vi "Main.vi"() -> ()   [LabVIEW 2013]
doc: "Use this template to build a simple state machine design pattern. Each state executes code and determines which state to transition to."
uses:
  controls/MainState.ctl
  controls/MainData.ctl
  <vilib>/Utility/file.llb/Read From Spreadsheet File (DBL).vi
panel:
  out "File Path":path
  in  "Binner":bool
  in  "Iteration Start":bool
  in  "Iteration Pause":bool
  in  "Program Stop":bool
  in  "Settings":bool
  in  "Open":bool
  out "Error Chart":dbl(graph)
  out "Spectral Signal":cluster{"X":dbl, "Y":dbl}[](graph)
  out "Temporal Signal":cluster{"X":dbl, "Y":dbl}[](graph)
  out "Retrieved Trace":dbl[][](graph)
  out "Original Trace":dbl[][](graph)
  # "These controls have associated \"Value Changed\" events configured in the Event Structure on the diagram.\n\nReplace them (and reconfigure the Event Structure) with the controls you need for your application."
  # "This template is for the Simple State Machine design pattern.\n\nSee the block diagram for more information on how to use this template."
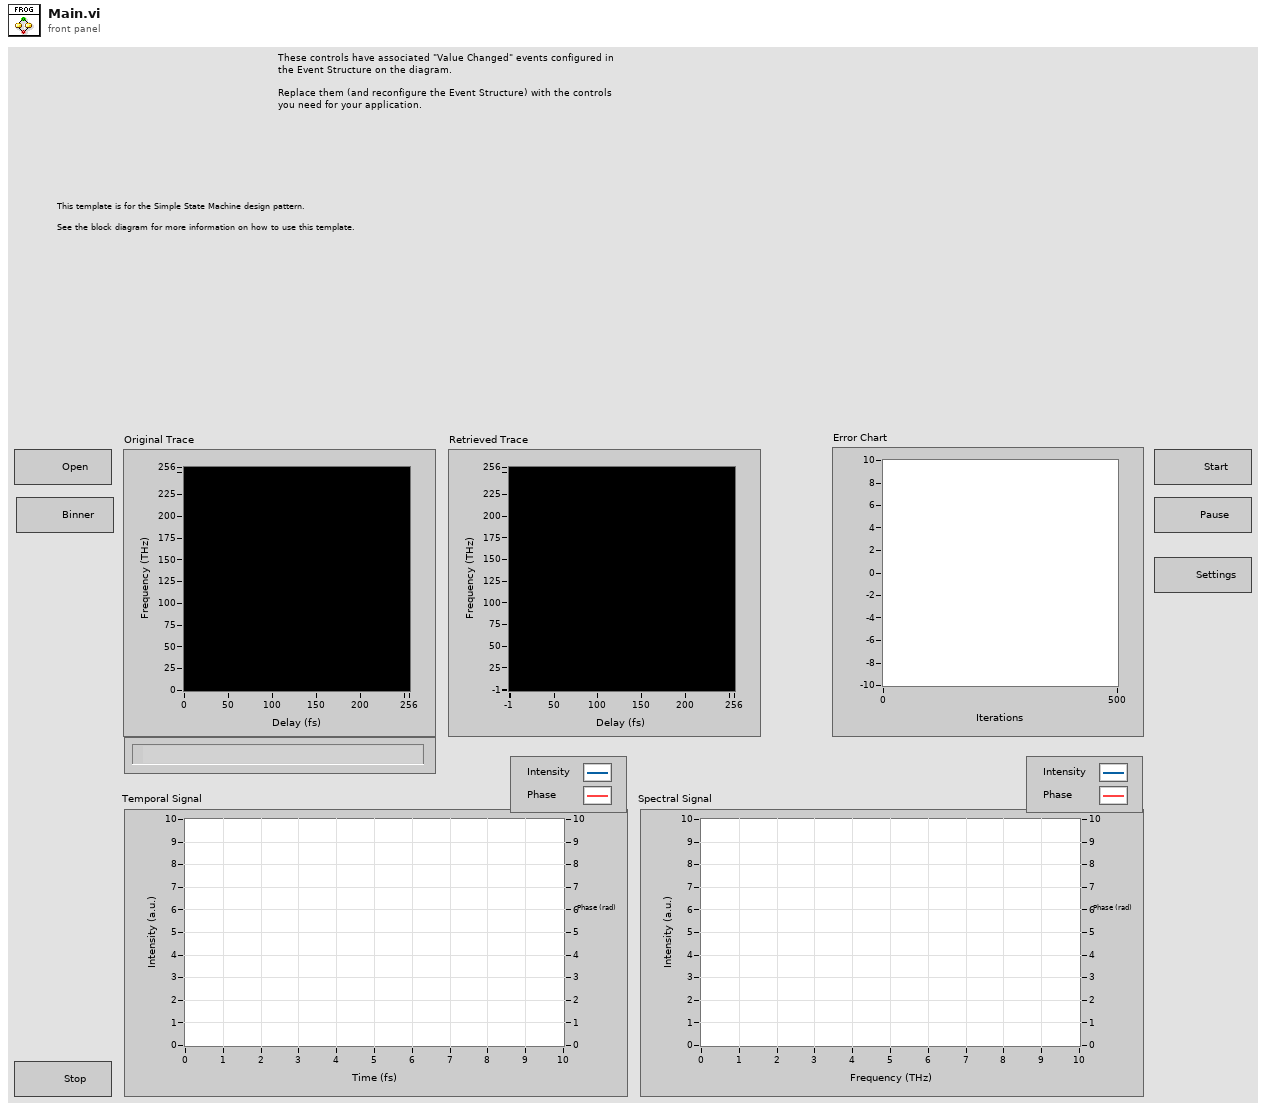
[diagram p1: front panel]
types:
  T1 = typedef "MainData.ctl" = cluster{"Template Trace":dbl[][], "Retrieved Trace":cdb[][], "Spectrum Info":cluster{"Frequency Max":dbl, "Frequency Min":dbl, "Spectrum Resolution":u16}, "Delay Info":cluster{"Temporal Resolution":u16, "Spatial Resolution":u16}, "RAW Trace":dbl[][]}
  T2 = typedef "MainState.ctl" = enum16{"Scale Changed", "Initialize", "Wait for Event", "Load File", "Start Retrieval", "Settings", "Binner", "Exit"}
  T3 = typedef "LVRangeTypeDef.ctl" = cluster{"Minimum":dbl, "Maximum":dbl, "Increment":dbl, "Minor Increment":dbl, "Start":dbl}
  T4 = cluster{"Delay Temporal Resolution":u16, "Delay Spatial Resolution":u16}
  T5 = cluster{"Frequency Max":dbl, "Frequency Min":dbl, "Spectrum Resolution":u16}
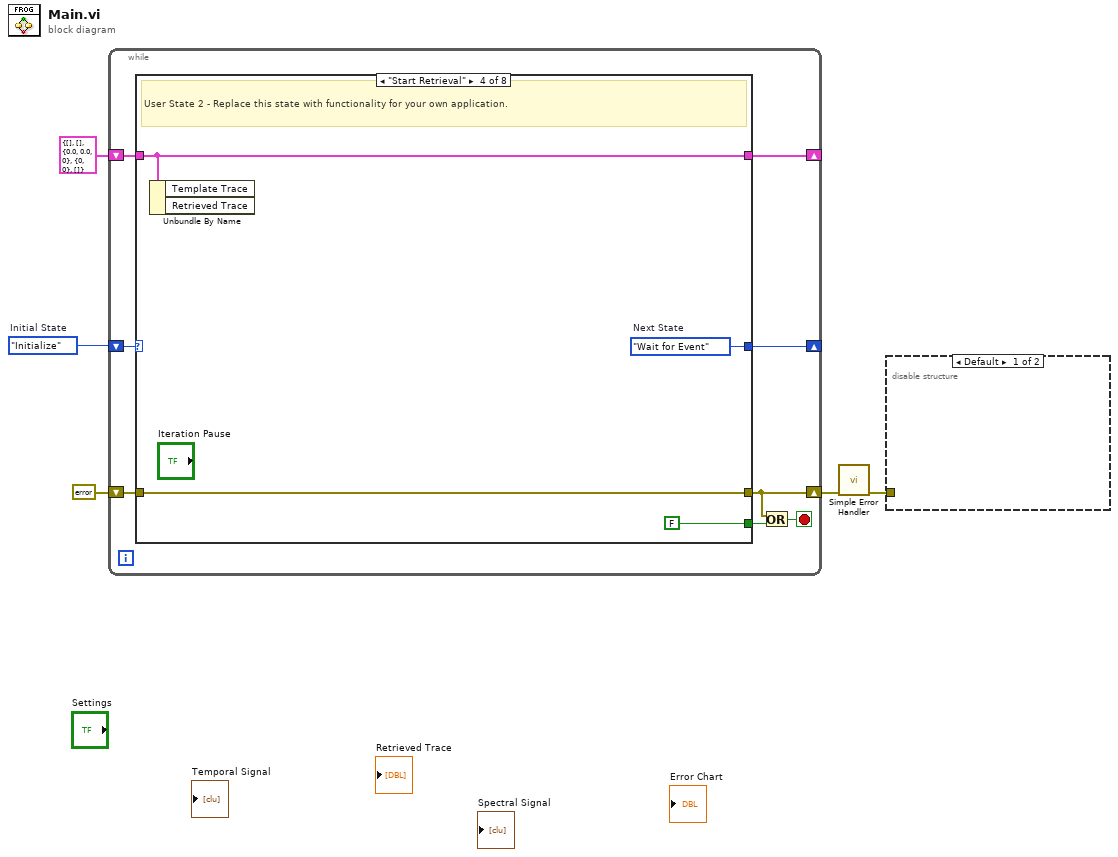
[diagram p0: block diagram]
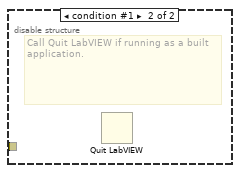
[diagram p2: hidden frame]
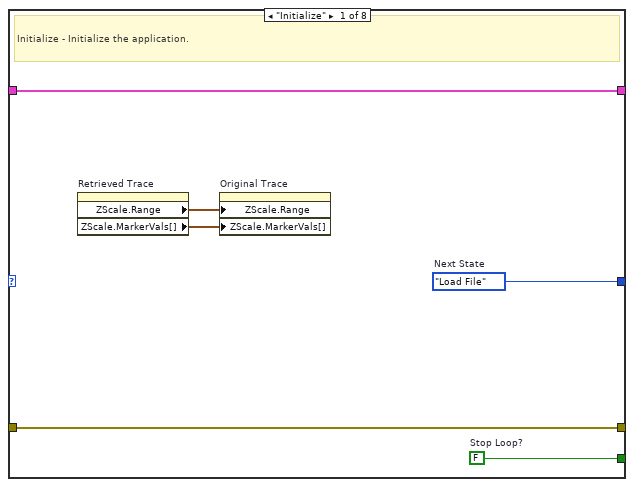
[diagram p3: hidden frame]
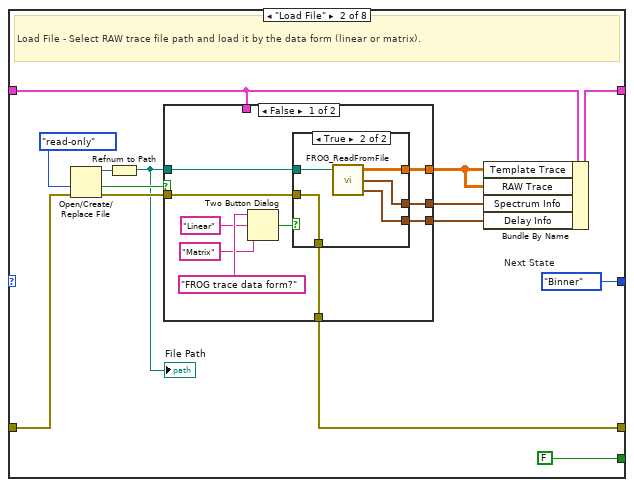
[diagram p4: hidden frame]
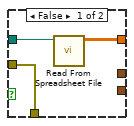
[diagram p5: hidden frame]
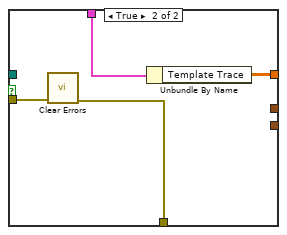
[diagram p6: hidden frame]
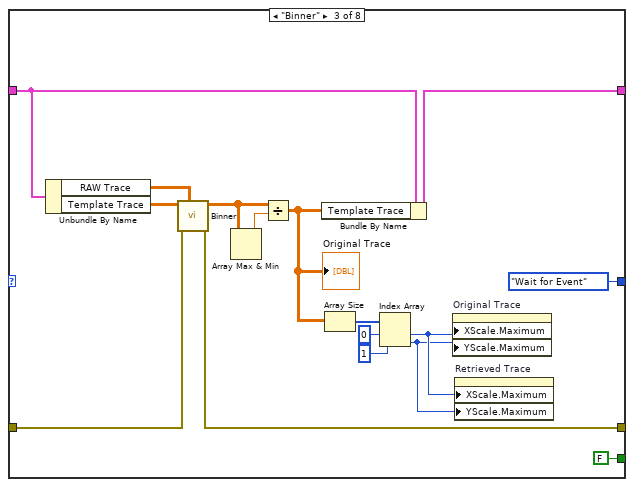
[diagram p7: hidden frame]
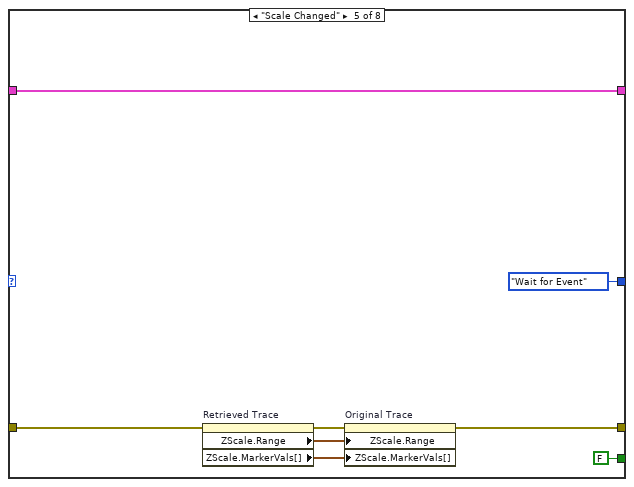
[diagram p8: hidden frame]
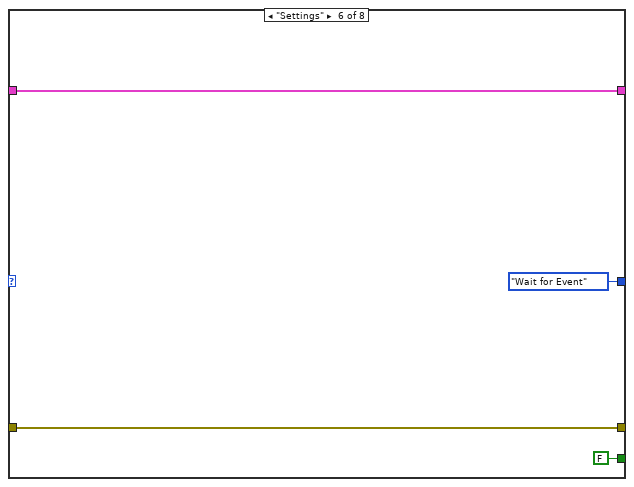
[diagram p9: hidden frame]
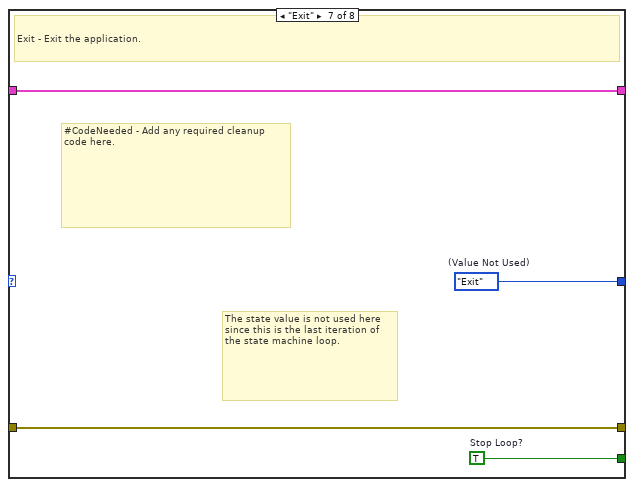
[diagram p10: hidden frame]
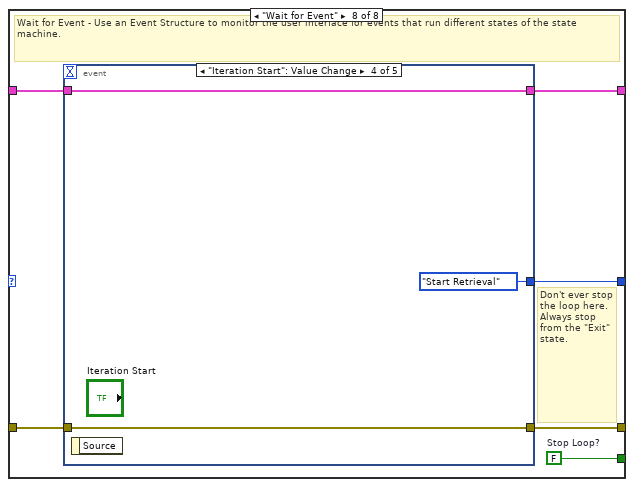
[diagram p11: hidden frame]
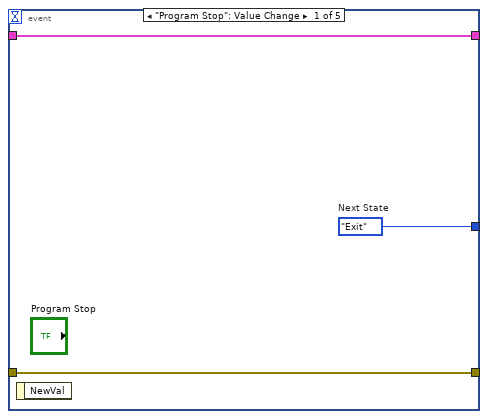
[diagram p12: hidden frame]
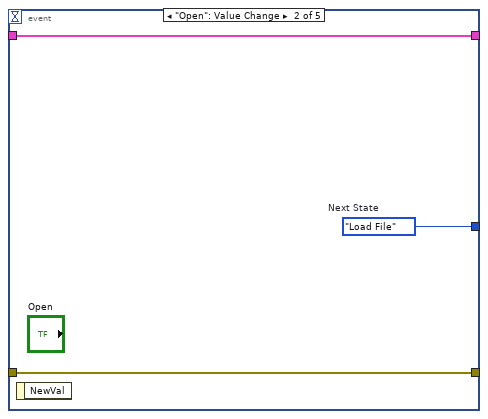
[diagram p13: hidden frame]
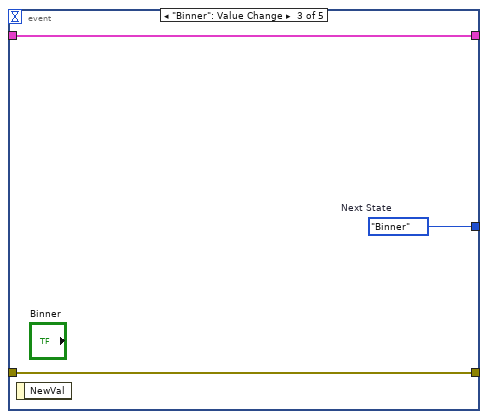
[diagram p14: hidden frame]
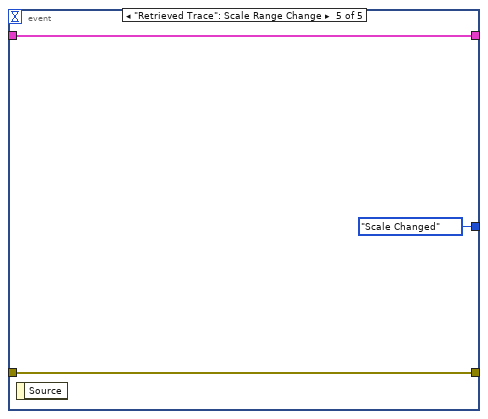
[diagram p15: hidden frame]
diagram:
  w5 = MainState."Initialize"  # Initial State
  n1 = while {
    shift-right: [w12] -> _
    shift-left: w5 -> [w13]
    shift-right: [w10] -> _
    shift-left: T1 {"Template Trace"=[], "Retrieved Trace"=[], "Spectrum Info"={"Frequency Max"=0.0, "Frequency Min"=0.0, "Spectrum Resolution"=0}, "Delay Info"={"Temporal Resolution"=0, "Spatial Resolution"=0}, "RAW Trace"=[]} ("Data") -> [w11]
    shift-right: [w6] -> w2
    shift-left: errorcluster {"status"=FALSE, "code"=0, "source"=""} ("error constant") -> [w9]
    stop <- w7 stop-if-true
    # "Main VI State Machine"
    n2 = case shown="\"Start Retrieval\"" w13 {
      tunnel: [w19 w33 MainState."Wait for Event" ("(Value Not Used)") w75 MainState."Wait for Event" ("Next State") MainState."Wait for Event" ("(Value Not Used)") w91 w97] -> w12
      tunnel: [w18 FALSE ("Stop Loop?") FALSE ("Stop Loop?") FALSE ("Stop Loop?") FALSE ("Stop Loop?") FALSE ("Stop Loop?") w89 w96] -> w8
      tunnel: w11 -> [w14 w24 w66 w72 w83 w87 w90 w95]
      tunnel: [w14 w27 w65 w72 w83 w87 w90 w94] -> w10
      tunnel: w9 -> [w17 w31 w69 w73 w80 w86 w88 w93]
      tunnel: [w17 w26 w68 w73 w78 w86 w88 w92] -> w6
      frame "Initialize" {
        w18 = FALSE  # Stop Loop?
        w19 = MainState."Load File"  # Next State
        # "Initialize - Initialize the application."
        n3 = property on="Retrieved Trace" class="IntGraph (strict)"() -> ("ZScale.Range"=w16:T3, "ZScale.MarkerVals[]"=w15:cluster{dbl, u32}[])  [unwired: 2 in, 2 out]
        n4 = property on="Original Trace" class="IntGraph (strict)"("ZScale.Range"=w16, "ZScale.MarkerVals[]"=w15) -> ()  [unwired: 2 in, 2 out]
      }
      frame "Load File" {
        w33 = MainState."Binner"  # Next State
        # "Load File - Select RAW trace file path and load it by the data form (linear or matrix)."
        n5 = Open/Create/Replace File(error in=w31, access (0:read/write)=enum16{"read/write", "read-only", "write-only"}."read-only") -> (refnum out=w29:refnum<file>, cancelled=w25:bool, error out=w28:errorcluster)  [unwired: 4 in]
        n6 = Refnum to Path(1:w29) -> (0:w23:path)
        "File Path" <- w23
        n7 = case shown="False" w25 {
          tunnel: w23 -> [w43 _]
          tunnel: w28 -> [w38 w55]
          tunnel: [w37 w52] -> w22
          tunnel: [w36 w54] -> w26
          tunnel: w24 -> [_ w53]
          tunnel: [w35 _] -> w21
          tunnel: [w34 _] -> w20
          frame False {
            n8 = Two Button Dialog(message="FROG trace data form?", 1:"Matrix" ("F button name (\"Cancel\")"), 2:"Linear" ("T button name (\"OK\")")) -> (T button?=w42:bool)
            n9 = case shown="True" w42 {
              tunnel: w43 -> [w45 w50]
              tunnel: [w46 w49] -> w37
              tunnel: w38 -> [w44 w51]
              tunnel: [w44 w51] -> w36
              tunnel: [_ w48] -> w35
              tunnel: [_ w47] -> w34
              frame False {
                n10 = call-poly <vilib>:"Read From Spreadsheet File.vi"("file path (dialog if empty)"=w45) -> ("all rows"=w46:dbl[][])  [unwired: 6 in, 4 out]
              }
              frame True {
                n11 = call "FROG_ReadFromFile.vi"("File Path"=w50) -> ("Delay Info"=w47:T4, "Spectrum Info"=w48:T5, "Experiment Trace"=w49:dbl[][])  [unwired: 2 in]
              }
            }
          }
          frame True {
            n12 = call <vilib>:"Clear Errors.vi"("error in (no error)"=w55) -> ("error out"=w54:errorcluster)  [unwired: 6 in]
            n13 = Unbundle By Name(w53) -> ("Template Trace"=w52:dbl[][])
          }
        }
        n14 = Bundle By Name(cluster=w24, "Template Trace"=w22, "RAW Trace"=w22, "Spectrum Info"=w21, "Delay Info"=w20) -> (w27:T1)
      }
      frame "Binner" {
        n15 = Unbundle By Name(w66) -> ("RAW Trace"=w64:dbl[][], "Template Trace"=w67:dbl[][])
        n16 = call "Binner.vi"("Default"=w64, "error in"=w69, "RAW Trace"=w67) -> ("error out"=w68:errorcluster, "Processed Trace"=w57:dbl[][])  [unwired: 2 in, 2 out]
        n17 = Array Max & Min(array=w57) -> (max value=w58:dbl)  [unwired: 3 out]
        n18 = Divide(x=w57, y=w58) -> (x/y=w56:dbl[][])
        "Original Trace" <- w56
        n19 = Bundle By Name(cluster=w66, "Template Trace"=w56) -> (w65:T1)
        n20 = Array Size(array=w56) -> (size(s)=w63:i32[])
        n21 = Index Array(array=w63, index #1=0 ("index"), index #2=1 ("index")) -> (element #1=w60:i32, element #2=w59:i32)
        n22 = property on="Original Trace" class="IntGraph (strict)"("XScale.Maximum"=w60, "YScale.Maximum"=w59) -> ()  [unwired: 2 in, 2 out]
        n23 = property on="Retrieved Trace" class="IntGraph (strict)"("XScale.Maximum"=w60, "YScale.Maximum"=w59) -> ()  [unwired: 2 in, 2 out]
      }
      frame "Start Retrieval" {
        w75 = MainState."Wait for Event"  # Next State
        # "User State 2 - Replace this state with functionality for your own application."
        n24 = Unbundle By Name(w72) -> ()  [unwired: 2 out]
      }
      frame "Scale Changed" {
        n25 = property on="Retrieved Trace" class="IntGraph (strict)"(error in=w80) -> (error out=w79:errorcluster, "ZScale.Range"=w82:T3, "ZScale.MarkerVals[]"=w81:cluster{dbl, u32}[])  [unwired: 1 in, 1 out]
        n26 = property on="Original Trace" class="IntGraph (strict)"(error in=w79, "ZScale.Range"=w82, "ZScale.MarkerVals[]"=w81) -> (error out=w78:errorcluster)  [unwired: 1 in, 1 out]
      }
      frame "Settings" {
      }
      frame "Exit" {
        w89 = TRUE  # Stop Loop?
        w91 = MainState."Exit"  # (Value Not Used)
        # "#CodeNeeded - Add any required cleanup code here."
        # "The state value is not used here since this is the last iteration of the state machine loop."
        # "Exit - Exit the application."
      }
      frame "Wait for Event" {
        w96 = FALSE  # Stop Loop?
        # "Don't ever stop the loop here. Always stop from the \"Exit\" state."
        # "Wait for Event - Use an Event Structure to monitor the user interface for events that run different states of the state machine."
        n27 = event shown="[3] \"Iteration Start\": Value Change" {
          selector: _ -> [_ _ _ _ _]
          dyn-events: _ -> [_ _ _ _ _]
          timeout: _ -> [_ _ _ _ _]
          tunnel: [w100 w103 w106 MainState."Start Retrieval" ("Next State") MainState."Scale Changed" ("Next State")] -> w97
          tunnel: w95 -> [w99 w101 w104 w109 w112]
          tunnel: [w99 w101 w104 w109 w112] -> w94
          tunnel: w93 -> [w98 w102 w105 w108 w111]
          tunnel: [w98 w102 w105 w108 w111] -> w92
          event "Program Stop": Value Change {
            w100 = MainState."Exit"  # Next State
            n28 = event-data() -> ()  [unwired: 1 in, 1 out]
          }
          event "Open": Value Change {
            w103 = MainState."Load File"  # Next State
            n29 = event-data() -> ()  [unwired: 1 in, 1 out]
          }
          event "Binner": Value Change {
            w106 = MainState."Binner"  # Next State
            n30 = event-data() -> ()  [unwired: 1 in, 1 out]
          }
          event "Iteration Start": Value Change {
            n31 = event-data() -> ()  [unwired: 1 in, 1 out]
          }
          event "Retrieved Trace": Scale Range Change {
            n32 = event-data() -> ()  [unwired: 1 in, 1 out]
          }
        }
      }
    }
    n33 = Or(x=w6, y=w8) -> (x .or. y?=w7:bool)
  }
  n34 = call <vilib>:"Simple Error Handler.vi"("error in (no error)"=w2) -> ("error out"=w1:errorcluster)  [unwired: 4 in, 4 out]
  n35 = disable-structure shown="Default" {
    disable-tunnel: w1 -> [_ _]
    frame condition #0 (active) {
    }
    frame condition #1 {
      # "Call Quit LabVIEW if running as a built application."
      n36 = Quit LabVIEW() -> ()  [unwired: 1 in]
    }
  }
